vi "CLASS - Display2DTest.vi"(8 "error in":errorcluster, 11 "Local":T6) -> (0 "error out":errorcluster, 3 "Local Out":T6)   [LabVIEW 2020]
doc: "Display the predicted data"
uses:
  Controls/2DParameters.ctl
  _Controls/Datas.ctl
  _Controls/PointPropertyMultipleLabel.ctl
  _Controls/Style.ctl
  _Controls/2DData.ctl
types:
  T1 = typedef "2DParameters.ctl" = cluster{"Plot":refnum<vi>, "Data":T2, "Display":cluster{"Choice":enum16{"All", "Train", "Test"}, "Indexe":cluster{"X":i32, "Y":i32}}, "Property":T3}
  T2 = typedef "Datas.ctl" = cluster{"Split":cluster{"X Train":dbl[][], "X Test":dbl[][], "Y Train":dbl[][], "Y Test":dbl[][]}, "Predict":dbl[][]}
  T3 = typedef "PointPropertyMultipleLabel.ctl" = cluster{"Train Style":T4, "Test OK Style":T4, "Label Color":u32[], "Test NO OK":cluster{"Style":T4, "Color":u32}}
  T4 = typedef "Style.ctl" = enum16{"Empty circle", "Full circle", "Empty square", "Full square", "Cross"}
  T5 = typedef "2DData.ctl" = cluster{"Tag":i32, "X":dbl[], "Y":dbl[]}
  T6 = cluster{"Parameters":T1, "2D Array":cluster{"X":dbl[], "Y":dbl[]}[], "Rating 2D Array":T5[], "Point ID":cluster{"DataUse":enum16{"Dataset", "Train", "Test"}, "Color":u32}[], "GoodPredict":i32}
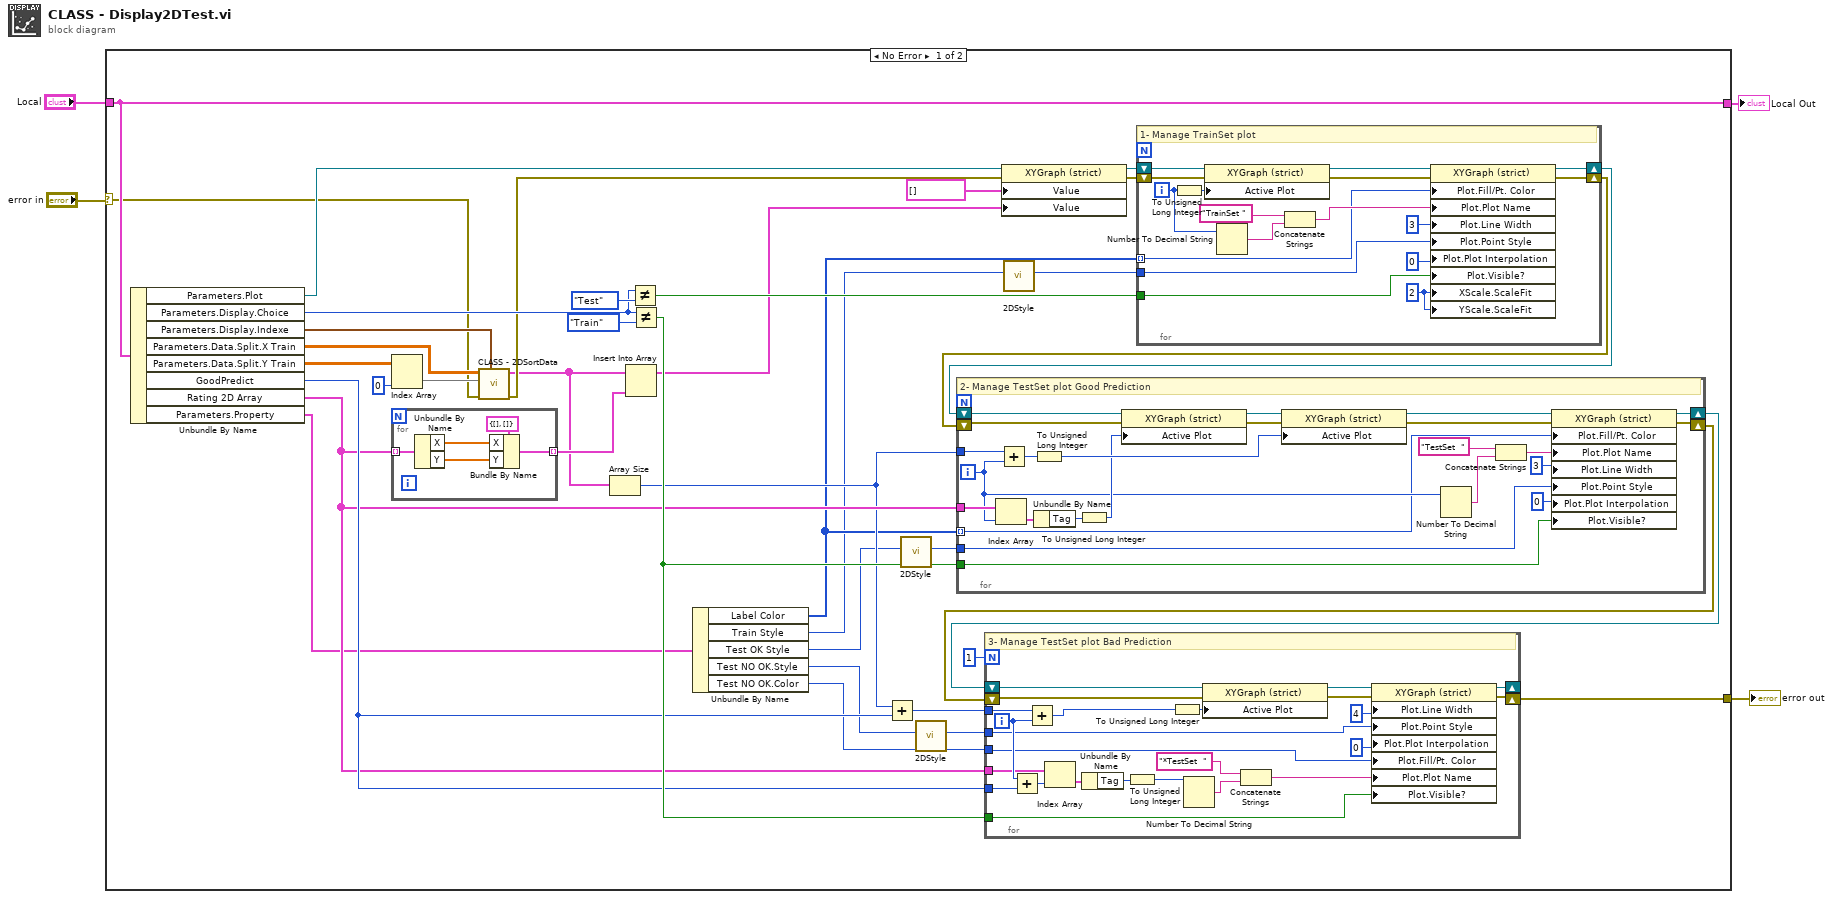
[diagram p0: block diagram]
diagram:
  n1 = case shown="No Error" "error in" {
    selector: "error in" -> [w17 w115]
    tunnel: [w19 w115] -> w3
    tunnel: "Local" -> [w26 w114]
    tunnel: [w26 w114] -> w1
    frame No Error {
      n2 = Unbundle By Name(w26) -> ("Parameters.Plot"=w30:refnum<vi>, "Parameters.Display.Choice"=w25:enum16{"All", "Train", "Test"}, "Parameters.Display.Indexe"=w18:cluster{"X":i32, "Y":i32}, "Parameters.Data.Split.X Train"=w24:dbl[][], "Parameters.Data.Split.Y Train"=w31:dbl[][], "GoodPredict"=w34:i32, "Rating 2D Array"=w33:T5[], "Parameters.Property"=w14:T3)
      n3 = Index Array(array=w31, index (col)=0 ("disabled index (col)")) -> (element=w21:dbl[])  [unwired: 1 in]
      n4 = for {
        tunnel: w33 -> [w113] mode=indexing
        tunnel: [w109] -> w38 mode=indexing
        n5 = Unbundle By Name(w113) -> ("X"=w111:dbl[], "Y"=w110:dbl[])
        n6 = Bundle By Name(cluster=cluster{"X":dbl[], "Y":dbl[]} {"X"=[], "Y"=[]} ("new element/subarray"), "X"=w111, "Y"=w110) -> (w109:cluster{"X":dbl[], "Y":dbl[]})
      }
      n7 = call "CLASS - 2DSortData.vi"("Index"=w18, "error in"=w17, "Y"=w21, "X"=w24) -> ("error out"=w23:errorcluster, "Array"=w22:cluster{"Array":dbl[], "Array":dbl[]}[])  [unwired: 6 in]
      n8 = Array Size(array=w22) -> (size(s)=w27:i32)
      n9 = Insert Into Array(array=w22, new element=w38) -> (w20:cluster{"Array":dbl[], "Array":dbl[]}[])  [unwired: 1 in]
      n10 = Not Equal?(x=w25, y=enum16{"All", "Train", "Test"}."Test") -> (x != y?=w36:bool)
      n11 = Not Equal?(x=w25, y=enum16{"All", "Train", "Test"}."Train") -> (x != y?=w35:bool)
      n12 = Unbundle By Name(w14) -> ("Label Color"=w13:u32[], "Train Style"=w10:T4, "Test OK Style"=w8:T4, "Test NO OK.Style"=w6:T4, "Test NO OK.Color"=w12:u32)
      n13 = Add(x=w27, y=w34) -> (x+y=w39:i32)
      n14 = call "2DStyle.vi"("Style"=w8) -> ("Style"=w7:u8)  [unwired: 10 in]
      n15 = call "2DStyle.vi"("Style"=w6) -> ("Style"=w5:u8)  [unwired: 10 in]
      n16 = property class="XYGraph (strict)"(reference=w30, error in=w23, "Value"=cluster{"X":dbl[], "Y":dbl[]}[] [], "Value"=w20) -> (reference out=w29:refnum<vi>, error out=w28:errorcluster)
      n17 = call "2DStyle.vi"("Style"=w10) -> ("Style"=w9:u8)  [unwired: 10 in]
      n18 = for {
        shift-right: [w50] -> w43
        shift-left: w28 -> [w59]
        shift-right: [w49] -> w42
        shift-left: w29 -> [w60]
        tunnel: w36 -> [w48]
        tunnel: w9 -> [w45]
        tunnel: w13 -> [w44] mode=indexing
        i -> [w52]
        w47 = u8 2 ("X Scale.Scale Fit")
        # "1- Manage TrainSet plot"
        n19 = To Unsigned Long Integer(number=w52) -> (unsigned 32bit integer=w58:u32)
        n20 = property class="XYGraph (strict)"(reference=w60, error in=w59, "Active Plot"=w58) -> (reference out=w57:refnum<vi>, error out=w56:errorcluster)
        n21 = Number To Decimal String(number=w52) -> (decimal integer string=w54:string)  [unwired: 1 in]
        n22 = Concatenate Strings("TrainSet " ("Plot.Plot Name"), w54) -> (w46:string)
        n23 = property class="XYGraph (strict)"(reference=w57, error in=w56, "Plot.Fill/Pt. Color"=w44, "Plot.Plot Name"=w46, "Plot.Line Width"=u8 3, "Plot.Point Style"=w45, "Plot.Plot Interpolation"=u8 0, "Plot.Visible?"=w48, "XScale.ScaleFit"=w47, "YScale.ScaleFit"=w47) -> (reference out=w49:refnum<vi>, error out=w50:errorcluster)
      }
      n24 = for {
        shift-right: [w70] -> w40
        shift-left: w43 -> [w71]
        shift-right: [w78] -> w41
        shift-left: w42 -> [w72]
        tunnel: w27 -> [w76]
        tunnel: w33 -> [w77]
        tunnel: w35 -> [w65]
        tunnel: w7 -> [w62]
        tunnel: w13 -> [w61] mode=indexing
        i -> [w68]
        # "2- Manage TestSet plot Good Prediction"
        n25 = Index Array(array=w77, index=w68) -> (element=w75:T5)
        n26 = Add(x=w76, y=w68) -> (x+y=w67:i32)
        n27 = To Unsigned Long Integer(number=w67) -> (unsigned 32bit integer=w84:u32)
        n28 = Unbundle By Name(w75) -> ("Tag"=w73:i32)
        n29 = To Unsigned Long Integer(number=w73) -> (unsigned 32bit integer=w74:u32)
        n30 = property class="XYGraph (strict)"(reference=w72, error in=w71, "Active Plot"=w74) -> (reference out=w64:refnum<vi>, error out=w63:errorcluster)
        n31 = property class="XYGraph (strict)"(reference=w64, error in=w63, "Active Plot"=w84) -> (reference out=w83:refnum<vi>, error out=w82:errorcluster)
        n32 = Number To Decimal String(number=w68) -> (decimal integer string=w80:string)  [unwired: 1 in]
        n33 = Concatenate Strings("TestSet  " ("Plot.Plot Name"), w80) -> (w66:string)
        n34 = property class="XYGraph (strict)"(reference=w83, error in=w82, "Plot.Fill/Pt. Color"=w61, "Plot.Plot Name"=w66, "Plot.Line Width"=u8 3, "Plot.Point Style"=w62, "Plot.Plot Interpolation"=u8 0, "Plot.Visible?"=w65) -> (reference out=w78:refnum<vi>, error out=w70:errorcluster)
      }
      n35 = for {
        N: 1 -> [_]
        shift-right: [w97] -> w19
        shift-left: w40 -> [w90]
        shift-right: [w102] -> _
        shift-left: w41 -> [w89]
        tunnel: w39 -> [w100]
        tunnel: w33 -> [w94]
        tunnel: w34 -> [w95]
        tunnel: w35 -> [w87]
        tunnel: w5 -> [w85]
        tunnel: w12 -> [w86]
        i -> [w96]
        # "3- Manage TestSet plot Bad Prediction"
        n36 = Add(x=w96, y=w95) -> (x+y=w93:i32)
        n37 = Add(x=w100, y=w96) -> (x+y=w101:i32)
        n38 = Index Array(array=w94, index=w93) -> (element=w99:T5)
        n39 = Unbundle By Name(w99) -> ("Tag"=w98:i32)
        n40 = To Unsigned Long Integer(number=w98) -> (unsigned 32bit integer=w91:u32)
        n41 = To Unsigned Long Integer(number=w101) -> (unsigned 32bit integer=w108:u32)
        n42 = Number To Decimal String(number=w91) -> (decimal integer string=w104:string)  [unwired: 1 in]
        n43 = property class="XYGraph (strict)"(reference=w89, error in=w90, "Active Plot"=w108) -> (reference out=w107:refnum<vi>, error out=w106:errorcluster)
        n44 = Concatenate Strings("*TestSet  " ("Plot.Plot Name"), w104) -> (w88:string)
        n45 = property class="XYGraph (strict)"(reference=w107, error in=w106, "Plot.Line Width"=u8 4, "Plot.Point Style"=w85, "Plot.Plot Interpolation"=u8 0, "Plot.Fill/Pt. Color"=w86, "Plot.Plot Name"=w88, "Plot.Visible?"=w87) -> (reference out=w102:refnum<vi>, error out=w97:errorcluster)
      }
    }
    frame Error {
    }
  }
  "error out" <- w3
  "Local Out" <- w1
